vi "Build Path.vi"(5 "Subroutine in":refnum<class "Subroutine.lvclass">, 6 "Path Builder":refnum<class "IPath Builder.lvclass">, 7 "Linked List ID":string, 8 "error in (no error)":errorcluster, 11 "Linked List Ref":refnum<data-value>) -> (0 "error out":errorcluster, 2 "Path":path, 3 "Linked List Ref out":refnum<data-value>)   [LabVIEW 2017, in "Custom Type Test Executive.lvlib" / "Subroutine.lvclass"]
uses:
  <vilib>/gpm_packages/@cs/test-executive/Source/Custom Type Test Executive/Subroutine/Subroutine.lvclass
  <vilib>/gpm_packages/@cs/linked-list/Source/Linked List/ILinkedList/ILinked List.lvclass
  <vilib>/gpm_packages/@cs/test-executive/Source/Path Builder/IPath Builder/IPath Builder.lvclass
  <vilib>/gpm_packages/@cs/data-type-serializer/source/String/String.lvclass/String.ctl
  888a9af0-6a9d-4290-98ca-e36b0c6a4dcd.vi
  <vilib>/gpm_packages/@cs/data-type-serializer/source/String/String.lvclass
  C:/Program Files/National Instruments/LabVIEW 2017/vi.lib/gpm_packages/@cs/data-type-serializer/source/Data Type/Data Type.lvclass
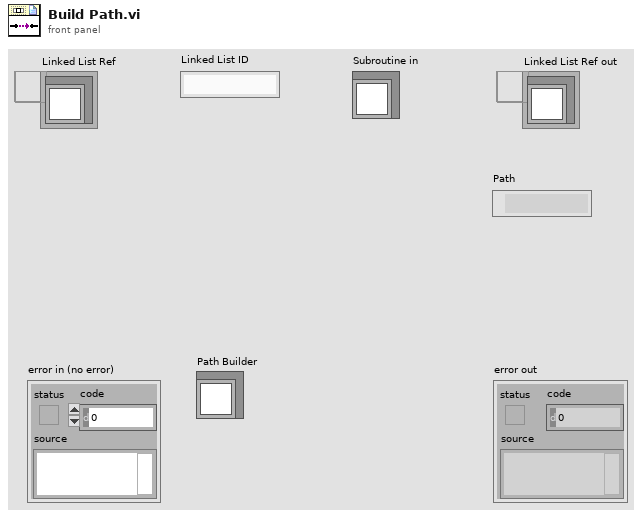
[diagram p1: front panel]
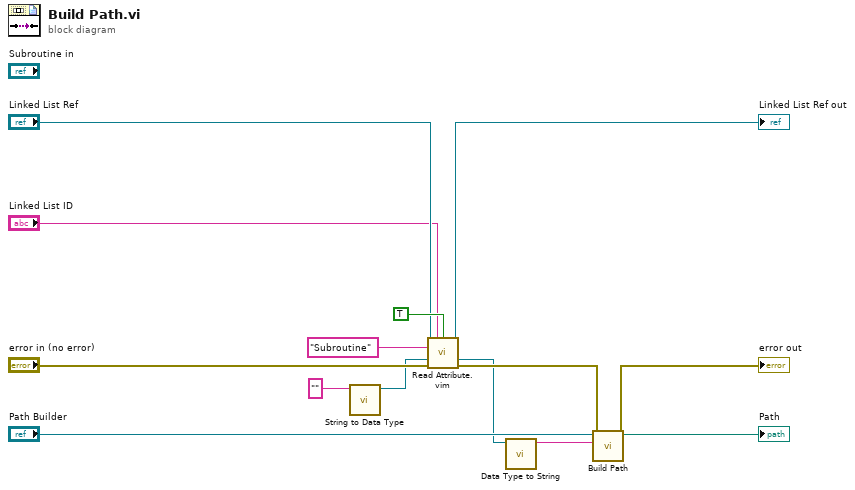
[diagram p0: block diagram]
diagram:
  n1 = call <vilib>:"String to Data Type.vi"("String"="") -> ("Boolean out"=w3:refnum<class "String.lvclass">)  [unwired: 9 in, 1 out]
  n2 = call "Read Attribute.vim"("Linked List Ref"="Linked List Ref", "Linked List ID"="Linked List ID", "Include Private?"=TRUE, "Attribute Name"="Subroutine", "Type"=w3, "error in (no error)"="error in (no error)") -> ("Linked List Ref out"=→"Linked List Ref out":refnum<data-value>, "Attribute"=w2:refnum<class "String.lvclass">, "error out"=w12:errorcluster)  [unwired: 4 in, 3 out]
  n3 = call <vilib>:"Data Type to String.vi"("Data Type"=w2) -> ("String out"=w1:string)  [unwired: 9 in, 1 out]
  n4 = call-dynamic "Build Path.vi"("error in (no error)"=w12, "Path"=w1, "IPath Builder in"="Path Builder") -> ("error out"=→"error out":errorcluster, "Path"=→"Path":path)  [unwired: 7 in]
